vi "Test Sclera.vi"() -> ()   [LabVIEW 2014]
uses:
  controls/Treatment Parameters.ctl
  controls/Results.ctl
  <vilib>/vision/NI_Vision_Development_Module.lvlib
panel:
  in  "error in (no error)":errorcluster
  out "Sclera Ratio":dbl
  out "Sclera Detected":bool
  out "Blue":T1 {"Standard  Variation" format="%.2f"; "Mean Value" format="%.2f"; "Interval Width" format="%.2f"; "Starting Value" format="%.2f"; "Maximal Value" format="%.2f"; "Minimal Value" format="%.2f"}
  out "Green":T1 {"Standard  Variation" format="%.2f"; "Mean Value" format="%.2f"; "Interval Width" format="%.2f"; "Starting Value" format="%.2f"; "Maximal Value" format="%.2f"; "Minimal Value" format="%.2f"}
  in  "Results":T2={"Center X"=500, "Center Y"=500, "Radius X"=150, "Radius Y"=0, "Score"=0, "Sclera Ratio"=0.0}
  in  "Treatment":T3={"Location"=50.0, "Width"=10.0, "Search"=enum."Lower"}
  out "Red":T1 {"Standard  Variation" format="%.2f"; "Mean Value" format="%.2f"; "Interval Width" format="%.2f"; "Starting Value" format="%.2f"; "Maximal Value" format="%.2f"; "Minimal Value" format="%.2f"}
  in  "Treatment Area Only":bool
  in  "File Path":path
  out "Image":T4(plugin-control)
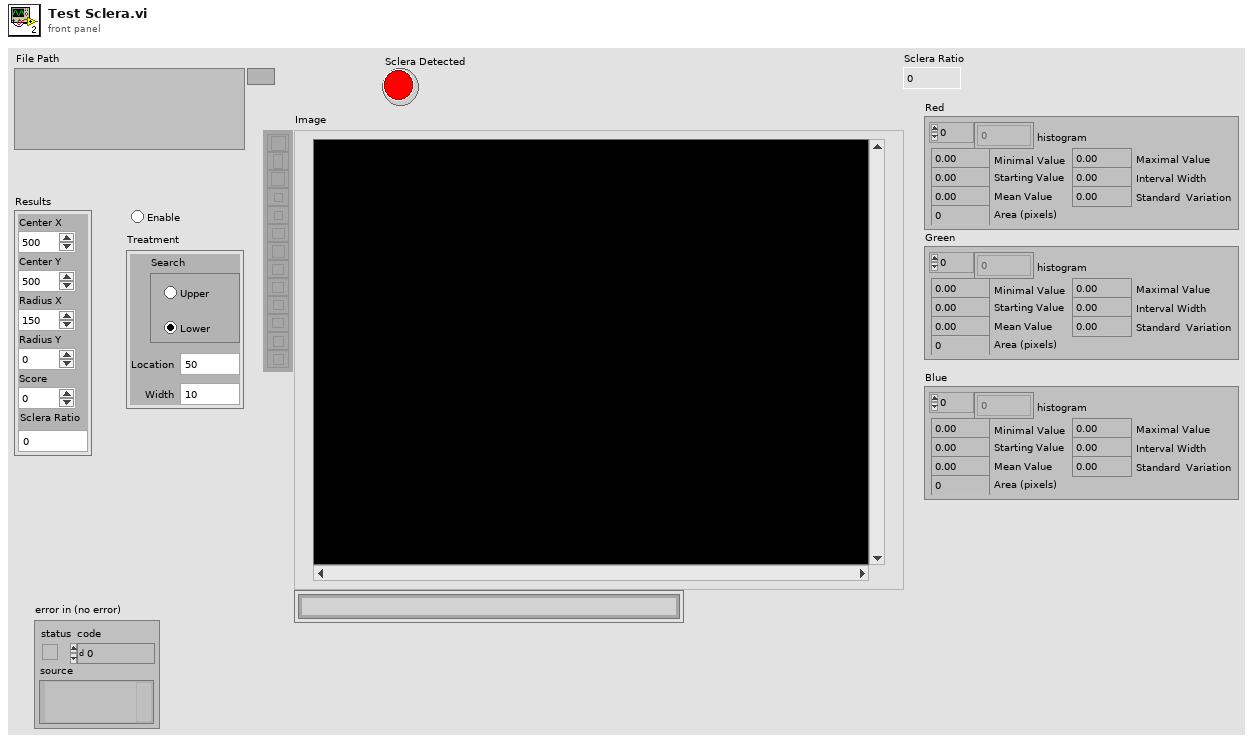
[diagram p1: front panel]
types:
  T1 = cluster{"histogram":u32[], "Minimal Value":sgl, "Maximal Value":sgl, "Starting Value":sgl, "Interval Width":sgl, "Mean Value":sgl, "Standard  Variation":sgl, "Area (pixels)":i32}
  T2 = typedef "Results.ctl" = cluster{"Center X":i32, "Center Y":i32, "Radius X":i32, "Radius Y":i32, "Score":i32, "Sclera Ratio":dbl}
  T3 = typedef "Treatment Parameters.ctl" = cluster{"Location":dbl, "Width":dbl, "Search":enum32{"Upper", "Lower"}}
  T4 = typedef "IMAQ Image.ctl" = refnum<image>
  T5 = typedef "Image Type" = u32
  T6 = typedef "ROI Descriptor" = cluster{"Global Rectangle":i32[], "Contours":cluster{"ID":enum32{"External", "Internal"}, "Type":u32, "Coordinates":i32[]}[]}
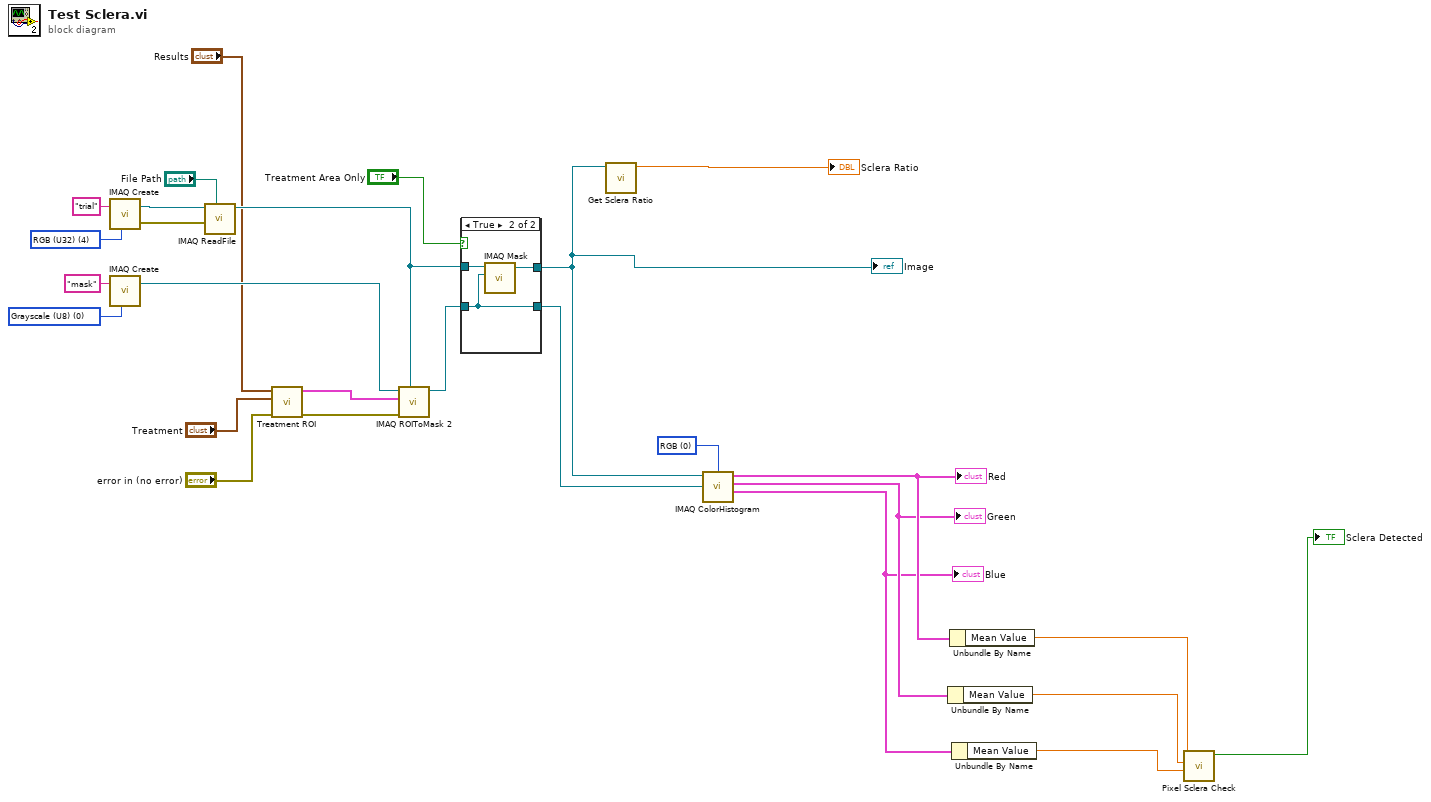
[diagram p0: block diagram]
diagram:
  w14 = u16 0 items=["RGB", "HSL", "HSV", "HSI", "CIE L*a*b*", "CIE XYZ"] ("Color Mode")
  w21 = T5 0 items=["Grayscale (U8)", "Grayscale (I16)", "Grayscale (SGL)", "Complex (CSG)", "RGB (U32)", "HSL (U32)", "RGB (U64)", "Grayscale (U16)"] ("Image Type")
  w22 = T5 4 items=["Grayscale (U8)", "Grayscale (I16)", "Grayscale (SGL)", "Complex (CSG)", "RGB (U32)", "HSL (U32)", "RGB (U64)", "Grayscale (U16)"] ("Image Type")
  n1 = call "IMAQ Create"("Image Name"="trial", "Image Type"=w22) -> ("New Image"=w27:T4, "error out"=w25:errorcluster)  [unwired: 3 in]
  n2 = call "IMAQ Create"("Image Name"="mask", "Image Type"=w21) -> ("New Image"=w19:T4)  [unwired: 3 in, 1 out]
  n3 = call "IMAQ ReadFile"("File Path"="File Path", "error in (no error)"=w25, "Image"=w27) -> ("Image Out"=w16:T4)  [unwired: 4 in, 4 out]
  n4 = call "Treatment ROI.vi"("error in (no error)"="error in (no error)", "Treatment"="Treatment", "Limbus"="Results") -> ("error out"=w17:errorcluster, "ROI Descriptor"=w23:T6)  [unwired: 7 in]
  n5 = call "IMAQ ROIToMask 2"("Image Model"=w16, "error in (no error)"=w17, "ROI Descriptor"=w23, "Image"=w19) -> ("Image Out"=w18:T4)  [unwired: 5 in, 2 out]
  n6 = case shown="True" "Treatment Area Only" {
    tunnel: w18 -> [w28 w30]
    tunnel: [w29 w32] -> w4
    tunnel: w16 -> [w29 w31]
    tunnel: [w28 w30] -> w2
    frame False {
    }
    frame True {
      n7 = call "IMAQ Mask"("Image Mask"=w30, "Image Src"=w31) -> ("Image Dst Out"=w32:T4)  [unwired: 3 in, 1 out]
    }
  }
  "Image" <- w4
  n8 = call "Get Sclera Ratio.vi"("Image"=w4) -> ("Sclera Ratio"=→"Sclera Ratio":dbl)  [unwired: 10 in]
  n9 = call "IMAQ ColorHistogram"("Color Mode"=w14, "Image Src"=w4, "Image Mask"=w2) -> ("Red or Hue or X or L* Histogram Report"=w11:T1, "Green or Sat or Y or a* Histogram Report"=w10:T1, "Blue or Luma or Val or Inten or Z or b* Histogram Report"=w9:T1)  [unwired: 3 in, 1 out]
  "Red" <- w11
  "Green" <- w10
  "Blue" <- w9
  n10 = Unbundle By Name(w10) -> ("Mean Value"=w7:sgl)
  n11 = Unbundle By Name(w11) -> ("Mean Value"=w8:sgl)
  n12 = Unbundle By Name(w9) -> ("Mean Value"=w6:sgl)
  n13 = call "Pixel Sclera Check.vi"("Blue"=w6, "Green"=w7, "Red"=w8) -> ("RGB Sclera"=→"Sclera Detected":bool)  [unwired: 8 in]
